vi "CoMP-S New AISAS Motors TwoCams.vi"(5 "Motion Code":string="\u0004", 6 "error in (no error)":errorcluster, 8 "steps/sec":u32=20, 9 "motor rotation":bool caption="motor direction", 10 "Steps":dbl=1.0, 11 "Motor selection":enum32{"Rotation", "Difuser ", "Objective Lens"}(radio)=enum."Difuser ") -> (1 "Estimated time [sec]":dbl, 2 "Read Buffer Out":string, 3 "device found":bool, 4 "error out":errorcluster)   [LabVIEW 2014]
panel:
  out "Read B in INT":u8
  in  "error in (no error) 2":errorcluster
  out "motor":string
  out "motor rotation 2":bool caption="motor direction"
  in  "bytes  to read":i32=1
  out "sec":ext
  out "Bytes Read":u32
  out "velocity":string
  out "rotation":string
  out "steps High B":string
  out "steps Low B":string="d"
  out "Device Description":string
  in  "Device Index":u32
  # "Time [sec]"
  # "roration motor - left - v smere  hod. ruciciek\n                       opt. rychlost 50steps/s"
  # "difuser - right - open difuser\n      6000 steps total\nCLOSE - LEFT\noptimal speed - 60steps/s\nMK+JR, 20140305 prevod 1:4.375"
  # "velocity = 730,88/steps.p.sec"
  # "left"
  # "Slow = 0"
  # "Fast = 365"
  # "OFFF objective lens klesaju hodnotyy"
  # "right"
  # "ON  ide smerom hore rychlost 60 zdravy stred"
  # "Rotation motor: smer left otaca filter modul doprava v pohlade smerom odspodu\nrychlost 10steps/s"
  # "Zmena od 28-MAR-2013, Jaro doplnil inteligentne snimace a vynovil elektroniku motorov.\nTeraz je poradie prikazu: vyber motora ->kod pohybu -> Dolny byte -> horny byte -> smer -> rychlost\nmotory dostali novy kod: DIFF=01, OBJ.LENS=02,ROT=03"
  # "Uprava 25-AUG-2013: OBJ. LENS=02\nDIFF = 01\nROTATION = 00\n!!!!"
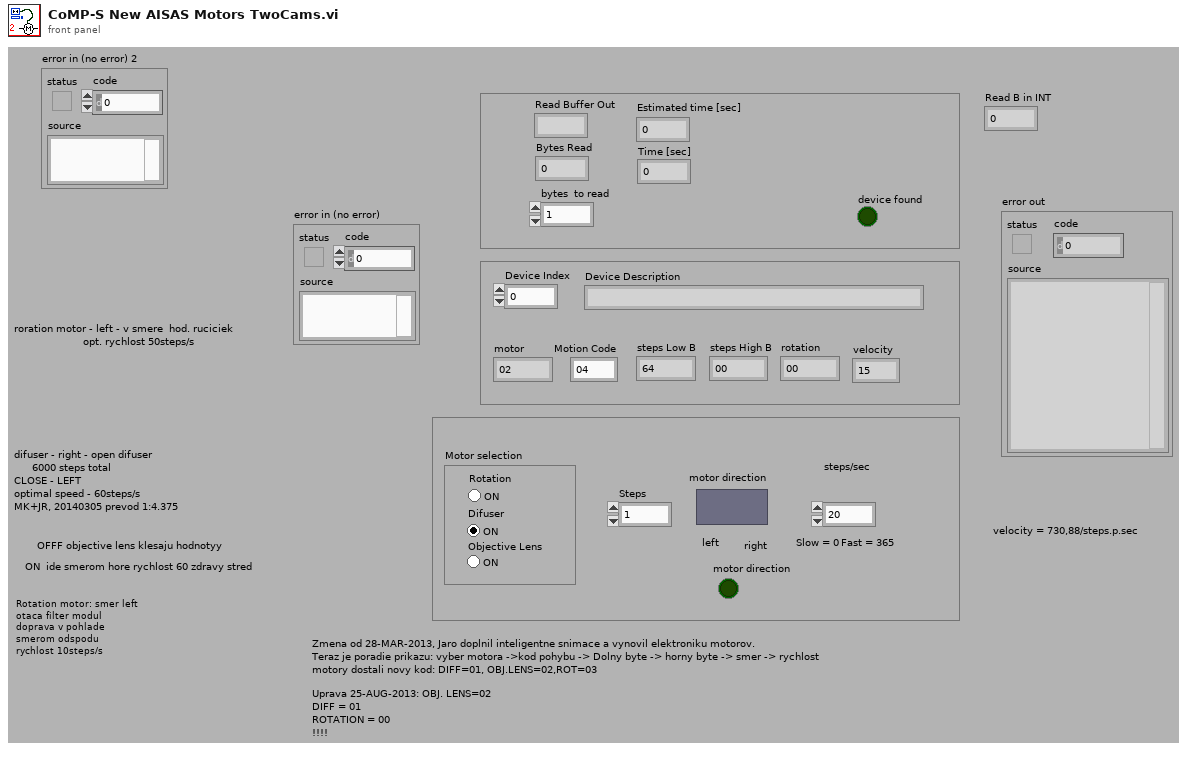
[diagram p1: front panel]
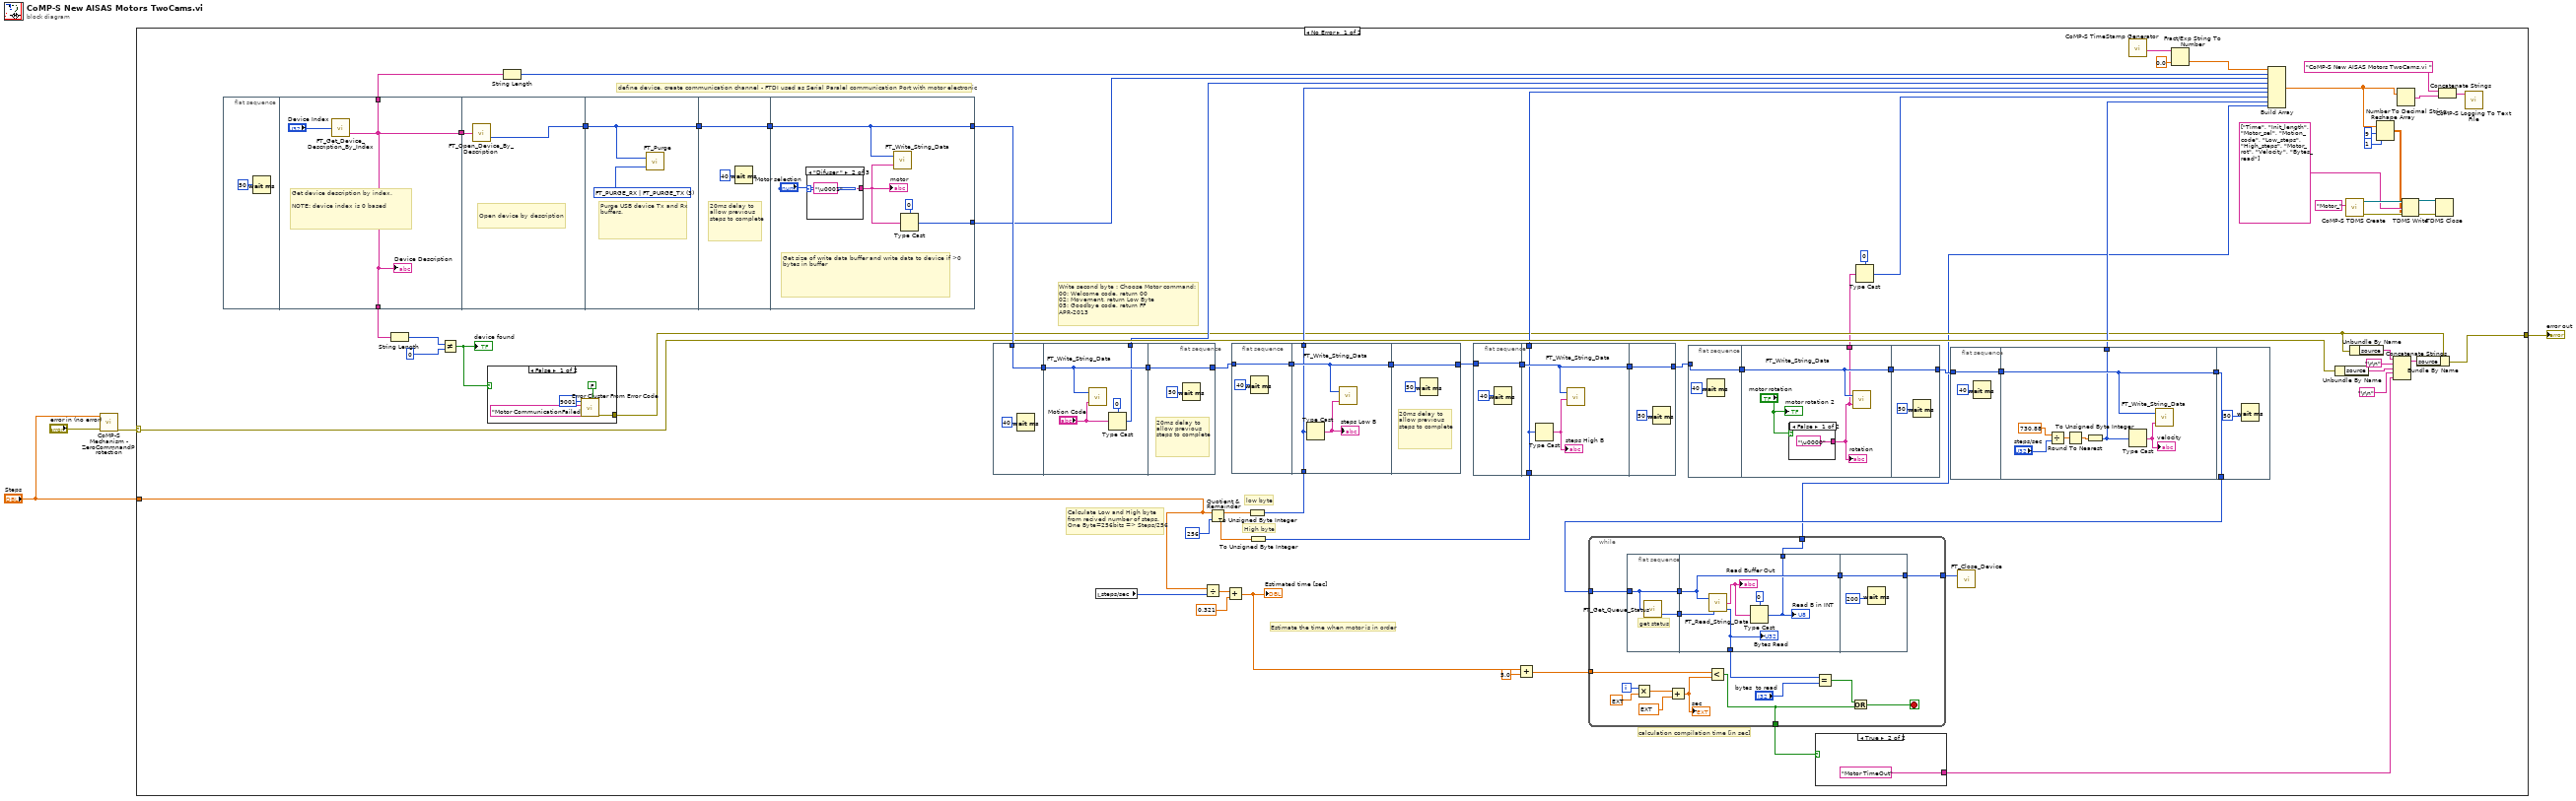
[diagram p0: block diagram]
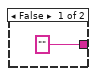
[diagram p2: hidden frame]
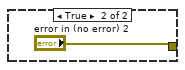
[diagram p3: hidden frame]
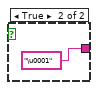
[diagram p4: hidden frame]
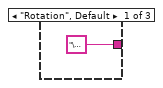
[diagram p5: hidden frame]
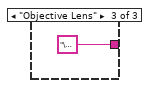
[diagram p6: hidden frame]
diagram:
  n1 = call "CoMP-S Mechanism - ZeroCommnandProtection.vi"("error in (no error)"="error in (no error)", "Arg 1"="Steps") -> ("error out"=w1:errorcluster)  [unwired: 9 in]
  n2 = case shown="No Error" w1 {
    selector: w1 -> [w36 w172]
    tunnel: [w40 w172] -> w4
    tunnel: "Steps" -> [w34 _]
    frame No Error {
      # "Estimate the time when motor is in order"
      # "Calculate Low and High byte\nfrom recived number of steps. \nOne Byte=256bits => Steps/256"
      # "Write second byte : Choose Motor command:\n00: Welcome code, return 00\n02: Movement, return Low Byte\n05: Goodbye code, return FF\nAPR-2013"
      # "define device, create communication channel - FTDI used as Serial Paralel communication Port with motor electronic"
      # "High byte"
      # "low byte"
      # "calculation compilation time [in sec]"
      n3 = flat-sequence {
        tunnel: [w156] -> w78
        tunnel: [w156] -> w50
        tunnel: [w156] -> w32
        tunnel: [w159] -> w77
        tunnel: w78 -> [w158]
        tunnel: [w160] -> w76
        tunnel: w77 -> [w160]
        tunnel: [w162] -> w75
        tunnel: w76 -> [w162]
        tunnel: [w168] -> w64
        tunnel: w75 -> [w168]
        tunnel: [w164] -> w30
        frame #0 {
          n4 = Wait (ms)(milliseconds to wait=u32 50) -> ()  [unwired: 1 out]
        }
        frame #1 {
          # "Get device description by index.\n\nNOTE: device index is 0 based"
          n5 = call "FT_Get_Device_Description_By_Index.vi"("Device Index"="Device Index") -> ("Device Description"=w156:string)  [unwired: 1 out]
          "Device Description" <- w156
        }
        frame #2 {
          # "Open device by description"
          n6 = call "FT_Open_Device_By_Description.vi"("Device Description"=w158) -> ("Handle"=w159:u32)  [unwired: 1 out]
        }
        frame #3 {
          w161 = u32 3 items=["FT_PURGE_RX"=1, "FT_PURGE_TX"=2, "FT_PURGE_RX | FT_PURGE_TX"=3] ("Purge Flags")
          # "Purge USB device Tx and Rx buffers."
          n7 = call "FT_Purge.vi"("Purge Flags"=w161, "Handle"=w160) -> ()  [unwired: 1 out]
        }
        frame #4 {
          # "20ms delay to allow previous steps to complete"
          n8 = Wait (ms)(milliseconds to wait=u32 40) -> ()  [unwired: 1 out]
        }
        frame #5 {
          # "Get size of write data buffer and write data to device if >0 bytes in buffer"
          n9 = case shown="\"Difuser \"" "Motor selection" {
            tunnel: ["\u0000" "\u0001" "\u0002"] -> w166
            frame "Rotation", Default {
            }
            frame "Difuser " {
            }
            frame "Objective Lens" {
            }
          }
          "motor" <- w166
          n10 = call "FT_Write_String_Data.vi"("Buffer"=w166, "Handle"=w168) -> ()  [unwired: 2 out]
          n11 = Type Cast(type=u8 0 ("default (0 U32)"), x=w166) -> (*(type *) &x=w164:u8)
        }
      }
      n12 = String Length(string=w50) -> (length=w49:i32)
      n13 = Not Equal?(x=w49, y=0) -> (x != y?=w47:bool)
      "device found" <- w47
      n14 = case shown="False" w47 {
        tunnel: [w81 "error in (no error) 2"] -> w19
        frame False {
          n15 = call <vilib>:"Error Cluster From Error Code.vi"("is warning? (False)"=FALSE, "error message (\"\")"="Motor CommunicationFailed" ("error message (\"\")"), "error code (0)"=9001) -> ("error out"=w81:errorcluster)  [unwired: 6 in]
        }
        frame True {
        }
      }
      n16 = String Length(string=w32) -> (length=w31:i32)
      n17 = flat-sequence {
        tunnel: [w148] -> w74
        tunnel: w64 -> [w148]
        tunnel: w74 -> [w152]
        tunnel: [w152] -> w73
        tunnel: [w149] -> w29
        tunnel: [w153] -> w63
        tunnel: w73 -> [w153]
        frame #0 {
          n18 = Wait (ms)(milliseconds to wait=u32 40) -> ()  [unwired: 1 out]
        }
        frame #1 {
          n19 = call "FT_Write_String_Data.vi"("Buffer"="Motion Code", "Handle"=w152) -> ()  [unwired: 2 out]
          n20 = Type Cast(type=u8 0 ("default (0 U32)"), x="Motion Code") -> (*(type *) &x=w149:u8)
        }
        frame #2 {
          # "20ms delay to allow previous steps to complete"
          n21 = Wait (ms)(milliseconds to wait=u32 50) -> ()  [unwired: 1 out]
        }
      }
      n22 = local read "steps/sec"() -> (w33:u32)
      n23 = Divide(x=w34, y=w33) -> (x/y=w52:dbl)
      n24 = Quotient & Remainder(x=w34, y=256) -> (x-y*floor(x/y)=w54:dbl, floor(x/y)=w56:dbl)
      n25 = Add(x=w52, y=0.321) -> (x+y=w45:dbl)
      "Estimated time [sec]" <- w45
      n26 = flat-sequence {
        tunnel: [w140] -> w72
        tunnel: w63 -> [w140]
        tunnel: [w144] -> w71
        tunnel: w53 -> [w142]
        tunnel: w72 -> [w144]
        tunnel: [w142] -> w28
        tunnel: [w145] -> w62
        tunnel: w71 -> [w145]
        frame #0 {
          n27 = Wait (ms)(milliseconds to wait=u32 40) -> ()  [unwired: 1 out]
        }
        frame #1 {
          n28 = Type Cast(x=w142) -> (*(type *) &x=w143:string)  [unwired: 1 in]
          "steps Low B" <- w143
          n29 = call "FT_Write_String_Data.vi"("Buffer"=w143, "Handle"=w144) -> ()  [unwired: 2 out]
        }
        frame #2 {
          # "20ms delay to allow previous steps to complete"
          n30 = Wait (ms)(milliseconds to wait=u32 50) -> ()  [unwired: 1 out]
        }
      }
      n31 = To Unsigned Byte Integer(number=w54) -> (unsigned 8bit integer=w53:u8)
      n32 = To Unsigned Byte Integer(number=w56) -> (unsigned 8bit integer=w55:u8)
      n33 = flat-sequence {
        tunnel: [w133] -> w70
        tunnel: w62 -> [w133]
        tunnel: [w137] -> w69
        tunnel: w55 -> [w135]
        tunnel: w70 -> [w137]
        tunnel: [w135] -> w27
        tunnel: [w138] -> w61
        tunnel: w69 -> [w138]
        frame #0 {
          n34 = Wait (ms)(milliseconds to wait=u32 40) -> ()  [unwired: 1 out]
        }
        frame #1 {
          n35 = Type Cast(x=w135) -> (*(type *) &x=w136:string)  [unwired: 1 in]
          "steps High B" <- w136
          n36 = call "FT_Write_String_Data.vi"("Buffer"=w136, "Handle"=w137) -> ()  [unwired: 2 out]
        }
        frame #2 {
          n37 = Wait (ms)(milliseconds to wait=u32 50) -> ()  [unwired: 1 out]
        }
      }
      n38 = Add(x=w45, y=5.0) -> (x+y=w44:dbl)
      n39 = while {
        tunnel: w59 -> [w102]
        tunnel: [w96] -> w58
        tunnel: w44 -> [w95]
        tunnel: [w87] -> w43
        tunnel: [w86] -> w9
        i -> [w90]
        stop <- w88 stop-if-true
        n40 = flat-sequence {
          tunnel: w102 -> [w103]
          tunnel: [w104] -> w101
          tunnel: [w103] -> w100
          tunnel: w101 -> [w110]
          tunnel: w100 -> [w108]
          tunnel: [w109] -> w98
          tunnel: [w108] -> w97
          tunnel: [w105] -> w86
          tunnel: w97 -> [w111]
          tunnel: [w111] -> w96
          frame #0 {
            # "get status"
            n41 = call "FT_Get_Queue_Status.vi"("Handle"=w103) -> ("Bytes Waiting"=w104:u32)  [unwired: 1 out]
          }
          frame #1 {
            n42 = call "FT_Read_String_Data.vi"("Handle"=w108, "Bytes To Read"=w110) -> ("Read Data"=w106:string, "Bytes Read"=w109:u32)  [unwired: 1 out]
            "Read Buffer Out" <- w106
            "Bytes Read" <- w109
            n43 = Type Cast(type=u8 0 ("default (0 U32)"), x=w106) -> (*(type *) &x=w105:u8)
            "Read B in INT" <- w105
          }
          frame #2 {
            n44 = Wait (ms)(milliseconds to wait=u32 200) -> ()  [unwired: 1 out]
          }
        }
        n45 = Multiply(x=w90, y=ext 0.2) -> (x*y=w93:ext)
        n46 = Add(x=w93, y=ext 0.32099999999999999999) -> (x+y=w89:ext)
        "sec" <- w89
        n47 = Less?(x=w95, y=w89) -> (x < y?=w87:bool)
        n48 = Equal?(x=w98, y="bytes  to read") -> (x = y?=w94:bool)
        n49 = Or(x=w94, y=w87) -> (x .or. y?=w88:bool)
      }
      n50 = flat-sequence {
        tunnel: [w125] -> w68
        tunnel: w61 -> [w125]
        tunnel: w68 -> [w128]
        tunnel: [w128] -> w67
        tunnel: [w126] -> w12
        tunnel: [w131] -> w60
        tunnel: w67 -> [w131]
        frame #0 {
          n51 = Wait (ms)(milliseconds to wait=u32 40) -> ()  [unwired: 1 out]
        }
        frame #1 {
          n52 = case shown="False" "motor rotation" {
            tunnel: ["\u0000" "\u0001"] -> w126
            frame False {
            }
            frame True {
            }
          }
          "rotation" <- w126
          n53 = call "FT_Write_String_Data.vi"("Buffer"=w126, "Handle"=w128) -> ()  [unwired: 2 out]
          "motor rotation 2" <- "motor rotation"
        }
        frame #2 {
          n54 = Wait (ms)(milliseconds to wait=u32 50) -> ()  [unwired: 1 out]
        }
      }
      n55 = case shown="True" w43 {
        tunnel: ["" "Motor TimeOut" ("error message (\"\")")] -> w38
        frame False {
        }
        frame True {
        }
      }
      n56 = Type Cast(type=u8 0 ("default (0 U32)"), x=w12) -> (*(type *) &x=w11:u8)
      n57 = flat-sequence {
        tunnel: [w113] -> w66
        tunnel: w60 -> [w113]
        tunnel: [w121] -> w65
        tunnel: w66 -> [w121]
        tunnel: [w115] -> w26
        tunnel: w65 -> [w122]
        tunnel: [w122] -> w59
        frame #0 {
          n58 = Wait (ms)(milliseconds to wait=u32 40) -> ()  [unwired: 1 out]
        }
        frame #1 {
          n59 = Divide(x=730.88, y="steps/sec") -> (x/y=w119:dbl)
          n60 = Round To Nearest(number=w119) -> (nearest integer value=w118:dbl)
          n61 = To Unsigned Byte Integer(number=w118) -> (unsigned 8bit integer=w115:u8)
          n62 = Type Cast(x=w115) -> (*(type *) &x=w120:string)  [unwired: 1 in]
          "velocity" <- w120
          n63 = call "FT_Write_String_Data.vi"("Buffer"=w120, "Handle"=w121) -> ()  [unwired: 2 out]
        }
        frame #2 {
          n64 = Wait (ms)(milliseconds to wait=u32 50) -> ()  [unwired: 1 out]
        }
      }
      n65 = call "FT_Close_Device.vi"("Handle"=w58) -> ()  [unwired: 1 out]
      n66 = call "CoMP-S TimeStamp Generator.vi"() -> ("date/time string"=w25:string)  [unwired: 10 in, 1 out]
      n67 = Fract/Exp String To Number(string=w25, default (0 dbl)=0.0 ("default (0 I32)")) -> (number=w23:dbl)  [unwired: 2 in, 1 out]
      n68 = Build Array(w23, w31, w30, w29, w28, w27, w11, w26, w9) -> (w8:dbl[])
      n69 = Unbundle By Name(w36) -> ("source"=w35:string)
      n70 = call "CoMP-S TDMS Create.vi"("Prefix"="Motor_") -> ("error out"=w20:errorcluster, "tdms file out"=w22:refnum<k34>)  [unwired: 7 in, 2 out]
      n71 = Unbundle By Name(w19) -> ("source"=w41:string)
      n72 = Reshape Array(w8, 9 ("dimension size"), 1 ("dimension size")) -> (w14:dbl[][])
      n73 = Concatenate Strings(w41, "\r\n", w35, "\r\n", w38) -> (w42:string)
      n74 = Number To Decimal String(number=w8) -> (decimal integer string=w7:string[])  [unwired: 1 in]
      n75 = TDMS Write(0:w22, 7:string[] ["Time", "Init_length", "Motor_sel", "Motion_code", "Low_steps", "High_steps", "Motor_rot", "Velocity", "Bytes_read"] ("initialized array"), 9:w14, 11:w20) -> (4:w17:refnum<k34>, 15:w18:errorcluster)  [unwired: 2 in, 2 out]
      n76 = Bundle By Name(cluster=w19, "source"=w42) -> (w40:errorcluster)
      n77 = TDMS Close(8:w18, 11:w17) -> ()  [unwired: 2 out]
      n78 = Concatenate Strings("CoMP-S New AISAS Motors TwoCams.vi " ("string"), w7) -> (w5:string)
      n79 = call "CoMP-S Logging To Text File.vi"("Input text"=w5) -> ()  [unwired: 10 in, 1 out]
    }
    frame Error {
    }
  }
  "error out" <- w4
